vi "Measurement Done.vi"(6 "Array of Hardware":refnum<class "Hardware.lvclass">[](array[class]), 8 "error in (no error)":errorcluster, 9 "Measurement Name":string, 10 "GUID":string, 11 "TestStand Controller in":refnum<class "Controller API.lvclass">) -> (0 "error out":errorcluster, 3 "TestStand Controller out":refnum<class "Controller API.lvclass">)   [LabVIEW 2015, in "Controller API.lvlib" / "Controller API.lvclass"]
uses:
  Controller API.lvclass
  <userlib>/Common Components/Hardware/Hardware.lvclass
  <userlib>/Common Components/Controller/Controller.lvclass
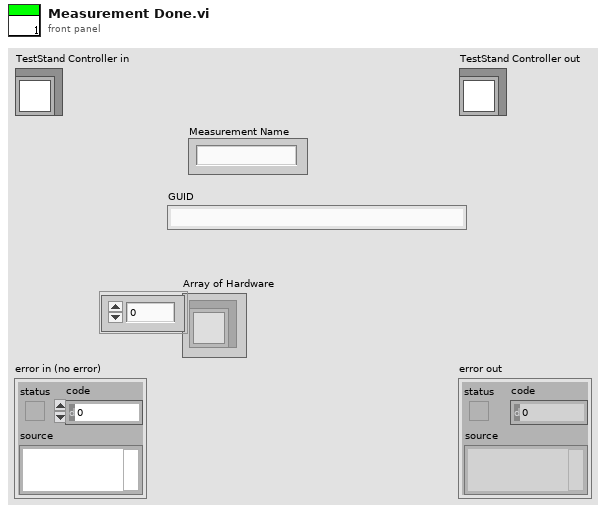
[diagram p1: front panel]
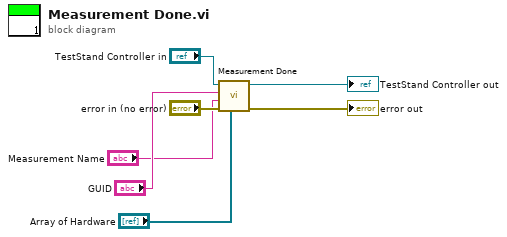
[diagram p0: block diagram]
diagram:
  n1 = call-parent "Measurement Done.vi"("Array of Hardware"="Array of Hardware", "error in (no error)"="error in (no error)", "Measurement Name"="Measurement Name", "GUID"="GUID", "Controller in"="TestStand Controller in") -> ("error out"=→"error out":errorcluster, "Controller out"=→"TestStand Controller out":refnum<class "Controller API.lvclass">)  [unwired: 5 in]
